vi "Actor Core.vi"(8 "error in":errorcluster, 11 "Launch IMAQ Display in":refnum<class "HIJ IMAQdx Camera Viewer.lvclass">) -> (0 "error out":errorcluster, 3 "Actor out":refnum<class "Actor.lvclass">)   [LabVIEW 2014, in "HIJ IMAQdx Justage Camera w Timer.lvlib" / "HIJ IMAQdx Camera Viewer.lvclass"]
doc: "(<B>Filename</B>: Actor Framework.lvlib:Actor.lvclass:Actor Core.vi)\n\nReceives messages to the actor, reacts to them, and initiates any error handling that may shut the actor down.\n\nDescendant classes may override this VI to append parallel tasks for the actor to complete while it handles messages. Overrides use the Call Parent Method node."
uses:
  HIJ IMAQdx Camera Viewer.lvclass
  <vilib>/ActorFramework/Actor/Actor.lvclass
  <vilib>/userdefined/High Color/IMAQdx.ctl
  Display Actors/HIJ IMAQdx Display/AF IMAQ Display/HIJ IMAQdx Display.lvclass
  Analyze/Analyze Classes/Analyze Diviation/Analyze BeamDeviation.lvclass
  Analyze/Results and Overlays/Results Beam Deviation/Analyze Results Beam Deviation.lvclass
  Analyze/Analyze Classes/Analyze Distanz/Analyze Distanz.lvclass
  Analyze/Results and Overlays/Results Distance/Analyze Results Distanz.lvclass
  Camera Actors/IMAQdx Actor/IMAQdx Actor/IMAQdx Actor.lvclass
  Display Actors/HIJ Vision Display/HIJ Vision Display/HIJ Vision Display.lvclass/HIJ Vision Display.ctl
  HIJ IMAQdx Camera Viewer.lvclass/HIJ IMAQdx Camera Viewer.ctl
  Applications/HIJ Vision Application/HIJ Vision Application/HIJ Vision Application.lvclass/HIJ Vision Application.ctl
  Applications/HIJ Vision Camera App/HIJ Vision Camera App/HIJ Vision Camera App.lvclass/HIJ Vision Camera App.ctl
  Shared Code/Viewable Actor/ViewableActor/ViewableActor.lvclass/ViewableActor.ctl
  <vilib>/ActorFramework/Actor/Actor.lvclass/Actor.ctl
  <vilib>/ActorFramework/Message Enqueuer/Message Enqueuer.lvclass/Message Enqueuer.ctl
  Applications/HIJ Vision Camera App/HIJ Vision Camera App Messages/Menu Selection Msg/Menu Selection Msg.lvclass/Menu Selection Msg.ctl
  Applications/HIJ Vision Application/HIJ Vision Application Messages/Write Image Prefix Msg/Write Image Prefix Msg.lvclass/Write Image Prefix Msg.ctl
  Applications/HIJ Vision Camera App/HIJ Vision Camera App Messages/Change Camera Msg/Change Camera Msg.lvclass/Change Camera Msg.ctl
  Display Actors/HIJ Vision Display/HIJ Vision Display/Write Save Report_.vi
  Applications/HIJ Vision Application/HIJ Vision Application/Write SubPnl for Display.vi
  Applications/HIJ Vision Camera App/HIJ Vision Camera App/Write Child Menu.vi
  Applications/HIJ Vision Application/HIJ Vision Application/Write HIJ Vision Display.vi
  Applications/HIJ Vision Application/HIJ Vision Application/Write Analyze Objs.vi
  Applications/HIJ Vision Camera App/HIJ Vision Camera App/Write Camera Actor.vi
  Shared Code/Viewable Actor/ViewableActor/Write UI VI Ref.vi
  <vilib>/ActorFramework/Message Enqueuer/Init from Existing Queue.vi
  <vilib>/ActorFramework/Message Enqueuer/Enqueue.vi
  Applications/HIJ Vision Camera App/HIJ Vision Camera App/Read Start Camera.vi
  <vilib>/ActorFramework/Message Priority Queue/Priority Enqueue.vi
  <vilib>/ActorFramework/Message Enqueuer/Message Enqueuer.lvclass
  Applications/HIJ Vision Camera App/HIJ Vision Camera App Messages/Menu Selection Msg/Menu Selection Msg.lvclass
  <vilib>/ActorFramework/Stop Msg/Stop Msg.lvclass
  Applications/HIJ Vision Application/HIJ Vision Application Messages/Write Image Prefix Msg/Write Image Prefix Msg.lvclass
  Applications/HIJ Vision Camera App/HIJ Vision Camera App Messages/Change Camera Msg/Change Camera Msg.lvclass
  Applications/HIJ Vision Application/HIJ Vision Application Messages/Save Image Msg/Save Image Msg.lvclass
  Applications/HIJ Vision Camera App/HIJ Vision Camera App/HIJ Vision Camera App.lvclass
panel:
  in  "Stop Button":bool
  in  "Camera":T1="TestCam"
  in  "Prefix":string
  in  "Save Button":bool
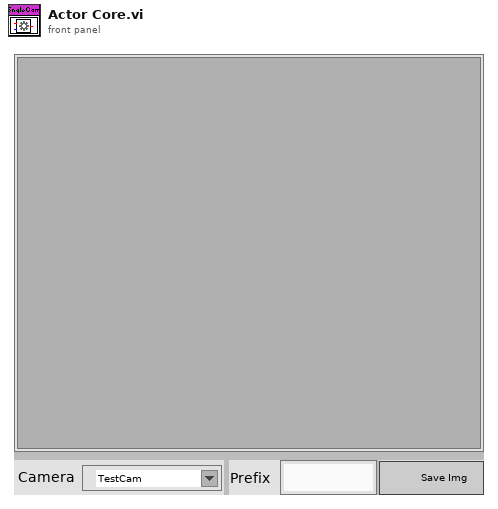
[diagram p1: front panel]
types:
  T1 = typedef "IMAQdx.ctl" = refnum<k21>
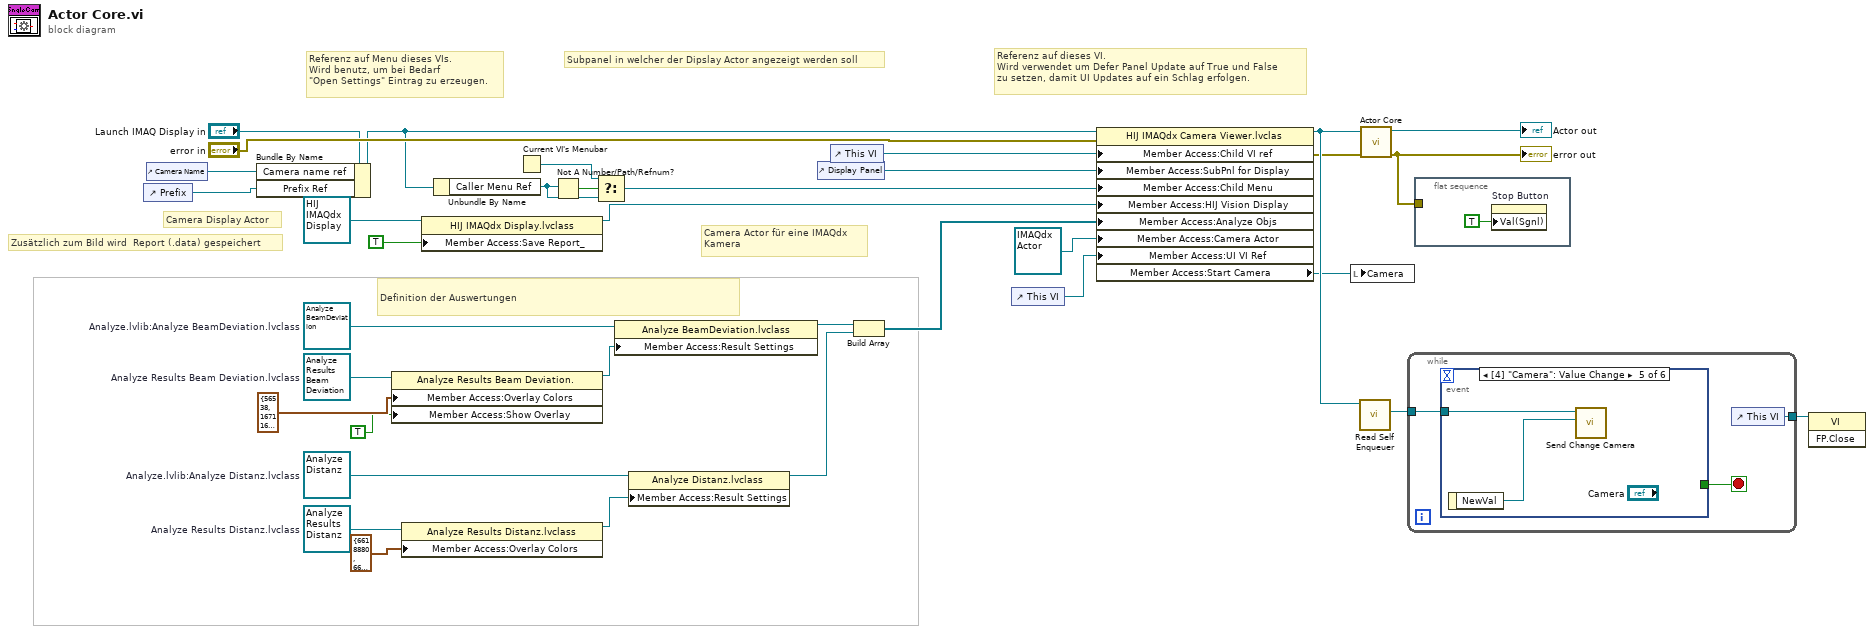
[diagram p0: block diagram]
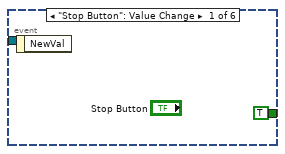
[diagram p2: hidden frame]
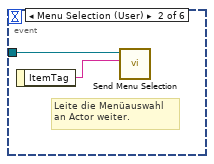
[diagram p3: hidden frame]
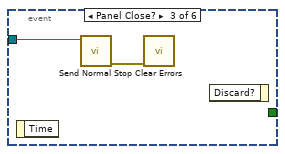
[diagram p4: hidden frame]
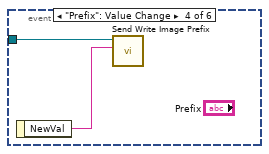
[diagram p5: hidden frame]
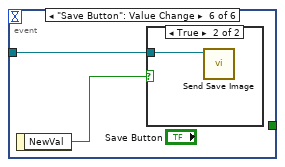
[diagram p6: hidden frame]
diagram:
  w26 = refnum<class "Analyze Results Distanz.lvclass"> refnum  # Analyze Results Distanz.lvclass
  w27 = refnum<class "Analyze Distanz.lvclass"> refnum  # Analyze.lvlib:Analyze Distanz.lvclass
  w29 = refnum<class "Analyze Results Beam Deviation.lvclass"> refnum  # Analyze Results Beam Deviation.lvclass
  w30 = refnum<class "Analyze BeamDeviation.lvclass"> refnum  # Analyze.lvlib:Analyze BeamDeviation.lvclass
  # "Camera Actor für eine IMAQdx\nKamera"
  # "Referenz auf Menu dieses VIs.\nWird benutz, um bei Bedarf \n\"Open Settings\" Eintrag zu erzeugen."
  # "Referenz auf dieses VI.\nWird verwendet um Defer Panel Update auf True und False\nzu setzen, damit UI Updates auf ein Schlag erfolgen."
  # "Definition der Auswertungen"
  # "Camera Display Actor"
  # "Zusätzlich zum Bild wird  Report (.data) gespeichert"
  # "Subpanel in welcher der Dipslay Actor angezeigt werden soll"
  n1 = control-ref of="Prefix"() -> (w2:refnum<vi>)
  n2 = control-ref of="Camera Name"() -> (w3:refnum<vi>)
  n3 = Bundle By Name(cluster="Launch IMAQ Display in", "Camera name ref"=w3, "Prefix Ref"=w2) -> (w4:refnum<class "HIJ IMAQdx Camera Viewer.lvclass">)
  n4 = property class="Analyze Results Beam Deviation."(reference=w29, "Member Access:Overlay Colors"=cluster{"Border":u32, "Text":u32} {"Border"=56538, "Text"=16711680} ("Colors"), "Member Access:Show Overlay"=TRUE ("Show Overlay")) -> (reference out=w15:refnum<class "Analyze Results Beam Deviation.lvclass">)  [unwired: 1 in, 1 out]
  n5 = property class="Analyze Results Distanz.lvclass"(reference=w26, "Member Access:Overlay Colors"=cluster{"Border":u32, "Text":u32} {"Border"=6618880, "Text"=6618880} ("Colors")) -> (reference out=w14:refnum<class "Analyze Results Distanz.lvclass">)  [unwired: 1 in, 1 out]
  n6 = property class="HIJ IMAQdx Display.lvclass"(reference=refnum<class "HIJ IMAQdx Display.lvclass"> refnum ("IMAQ Display.lvlib:IMAQ Display.lvclass"), "Member Access:Save Report_"=TRUE ("Save Report_")) -> (reference out=w17:refnum<class "HIJ IMAQdx Display.lvclass">)  [unwired: 1 in, 1 out]
  n7 = Unbundle By Name(w4) -> ("Caller Menu Ref"=w7:refnum<k9>)
  n8 = Current VI's Menubar() -> (w8:refnum<k9>)
  n9 = Not A Number/Path/Refnum?(number/path/refnum=w7) -> (NaN/Path/Refnum?=w10:bool)
  n10 = Select(t=w8, s=w10, f=w7) -> (s? t:f=w9:refnum<k9>)
  n11 = property class="Analyze BeamDeviation.lvclass"(reference=w30, "Member Access:Result Settings"=w15) -> (reference out=w16:refnum<class "Analyze BeamDeviation.lvclass">)  [unwired: 1 in, 1 out]
  n12 = property class="Analyze Distanz.lvclass"(reference=w27, "Member Access:Result Settings"=w14) -> (reference out=w13:refnum<class "Analyze Distanz.lvclass">)  [unwired: 1 in, 1 out]
  n13 = control-ref of="Display Panel"() -> (w19:refnum<vi>)
  n14 = control-ref of="This VI"() -> (w23:refnum<vi>)
  n15 = Build Array(w16, w13) -> (w20:refnum<class "Analyze BaseClass.lvclass">[])
  n16 = control-ref of="This VI"() -> (w12:refnum<vi>)
  n17 = property class="HIJ IMAQdx Camera Viewer.lvclas"(reference=w4, error in="error in", "Member Access:Child VI ref"=w23, "Member Access:SubPnl for Display"=w19, "Member Access:Child Menu"=w9, "Member Access:HIJ Vision Display"=w17, "Member Access:Analyze Objs"=w20, "Member Access:Camera Actor"=refnum<class "IMAQdx Actor.lvclass"> refnum ("IMAQdx Actor.lvlib:IMAQdx Actor.lvclass"), "Member Access:UI VI Ref"=w12) -> (reference out=w24:refnum<class "HIJ IMAQdx Camera Viewer.lvclass">, error out=w21:errorcluster, "Member Access:Start Camera"=w1:T1)
  n18 = local write "Camera"(w1) -> ()
  n19 = call <vilib>:"Read Self Enqueuer.vi"("Actor"=w24) -> ("Self Enqueuer"=w32:refnum<class "Message Enqueuer.lvclass">)  [unwired: 10 in]
  n20 = call-parent "Actor Core.vi"("error in"=w21, "HIJ Vision Camera App In"=w24) -> ("error out"=w33:errorcluster, "Actor out"=→"Actor out":refnum<class "Actor.lvclass">)  [unwired: 8 in]
  "error out" <- w33
  n21 = while {
    tunnel: w32 -> [w37]
    tunnel: [w36] -> w5
    stop <- w38 stop-if-true
    n22 = event shown="[4] \"Camera\": Value Change" {
      selector: _ -> [_ _ _ _ _ _]
      dyn-events: _ -> [_ _ _ _ _ _]
      timeout: _ -> [_ _ _ _ _ _]
      tunnel: [TRUE _ _ _ _ _] -> w38
      tunnel: w37 -> [_ w40 w43 w44 w47 w48]
      event "Stop Button": Value Change {
        n23 = event-data() -> ()  [unwired: 1 in, 1 out]
      }
      event Menu Selection (User) {
        # "Leite die Menüauswahl \nan Actor weiter."
        n24 = event-data() -> ("ItemTag"=w41:string)  [unwired: 1 in]
        n25 = call "Send Menu Selection.vi"("MenuTag"=w41, "Message Enqueuer"=w40) -> ()  [unwired: 8 in, 2 out]
      }
      event Panel Close? {
        n26 = event-data() -> ()  [unwired: 1 in, 1 out]
        n27 = call <vilib>:"Send Normal Stop.vi"("Message Enqueuer"=w43) -> ("error out"=w42:errorcluster)  [unwired: 10 in]
        n28 = call <vilib>:"Clear Errors.vi"("error in (no error)"=w42) -> ()  [unwired: 5 in, 2 out]
        n29 = event-data() -> ()  [unwired: 2 in, 1 out]
      }
      event "Prefix": Value Change {
        n30 = event-data() -> ("NewVal"=w45:string)  [unwired: 1 in]
        n31 = call "Send Write Image Prefix.vi"("Prefix"=w45, "Message Enqueuer"=w44) -> ()  [unwired: 8 in, 2 out]
      }
      event Value Change {
        n32 = event-data() -> ("NewVal"=w46:T1)  [unwired: 1 in]
        n33 = call "Send Change Camera.vi"("New Camera"=w46, "Message Enqueuer"=w47) -> ()  [unwired: 8 in, 2 out]
      }
      event "Save Button": Value Change {
        n34 = event-data() -> ("NewVal"=w49:bool)  [unwired: 1 in]
        n35 = case shown="True" w49 {
          tunnel: w48 -> [_ w50]
          frame False {
          }
          frame True {
            n36 = call "Send Save Image.vi"("Message Enqueuer"=w50) -> ()  [unwired: 9 in, 2 out]
          }
        }
      }
    }
    n37 = control-ref of="This VI"() -> (w36:refnum<vi>)
  }
  n38 = flat-sequence {
    tunnel: w33 -> [_]
    frame #0 {
      n39 = property on="Stop Button" class="Bool (strict)"("Val(Sgnl)"=TRUE) -> ()  [unwired: 2 in, 2 out]
    }
  }
  n40 = invoke class="VI" method="FP.Close"(reference=w5) -> ()  [unwired: 2 in, 3 out]
